vi "Read Tim Obs.vi"(8 "error in":errorcluster, 11 "tCRD in":refnum<class "tCRD.lvclass">) -> (0 "error out":errorcluster, 2 "Tim Obs":refnum<class "Tim File Observer.lvclass">, 3 "tCRD out":refnum<class "tCRD.lvclass">)   [LabVIEW 2015]
uses:
  tCRD.lvclass
  File Observer/Tim File Observer.lvclass
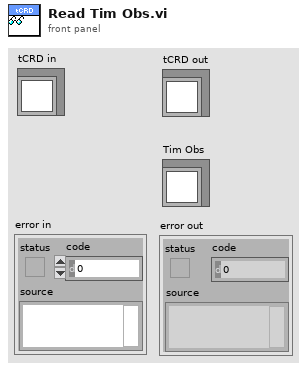
[diagram p1: front panel]
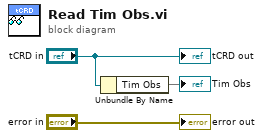
[diagram p0: block diagram]
diagram:
  n1 = Unbundle By Name("tCRD in") -> ("Tim Obs"=→"Tim Obs")
  "error out" <- "error in"
  "tCRD out" <- "tCRD in"
